vi "Convert Message Definition to Message Configuration.vi"(11 "message definition":T2={"name"="", "message type"="BC to RT", "endpoint Tx"={"terminal address"=0, "subaddress"=0}, "endpoint Rx"={"terminal address"=0, "subaddress"=0}, "create timestamp channel"=FALSE, "mode code"=0, "number of words"=0, "parameters"=[]}) -> (3 "message configuration":T1)   [LabVIEW 2020, in "AIM MIL-STD-1553 Engine.lvlib" / "Implementation.lvlib" / "Shared Resources Factory.lvclass"]
uses:
  Shared Resources Factory.lvclass
  Shared/Message Definition.ctl
  Shared/Message Type.ctl
  Shared/Terminal Endpoint.ctl
  Shared/Address.ctl
  Shared/Parameter Definition.ctl
  Custom Device/Message Configuration.ctl
  Custom Device/Custom Device.lvlib
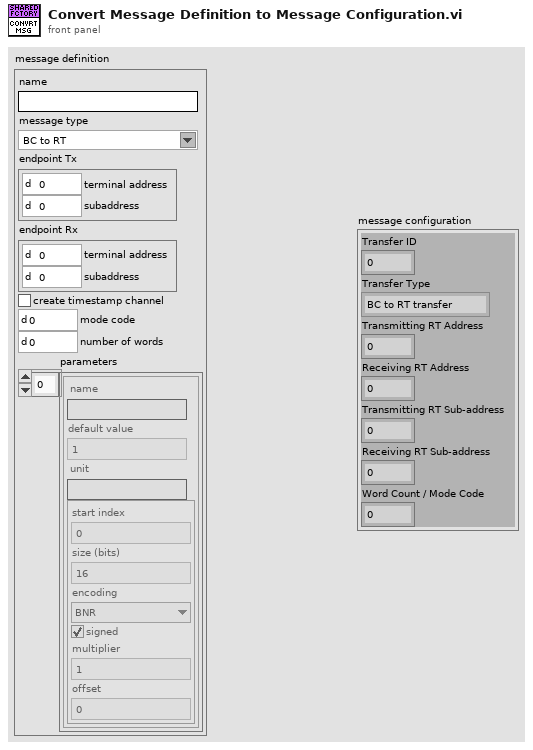
[diagram p1: front panel]
types:
  T1 = typedef "AIM MIL-STD-1553 Engine.lvlib/Custom Device.lvlib/Message Configuration.ctl" = cluster{"Transfer ID":u16, "Transfer Type":enum16{"BC to RT transfer", "RT to BC transfer", "RT to RT transfer"}, "Transmitting RT Address":u8, "Receiving RT Address":u8, "Transmitting RT Sub-address":u8, "Receiving RT Sub-address":u8, "Word Count / Mode Code":u8}
  T2 = typedef "Message Definition.ctl" = cluster{"name":string, "message type":T3, "endpoint Tx":T4, "endpoint Rx":T4, "create timestamp channel":bool, "mode code":u16, "number of words":u16, "parameters":cluster{"name":string, "default value":dbl, "unit":string, "parameter definition":T6}[]}
  T3 = typedef "Message Type.ctl" = string
  T4 = typedef "Terminal Endpoint.ctl" = cluster{"terminal address":T5, "subaddress":T5}
  T5 = typedef "Address.ctl" = u16
  T6 = typedef "Parameter Definition.ctl" = cluster{"start index":i32, "size (bits)":i32, "encoding":enum16{"BNR", "BCD", "Discrete"}, "signed":bool, "multiplier":dbl, "offset":dbl}
  T7 = enum16{"BC to RT transfer", "RT to BC transfer", "RT to RT transfer"}
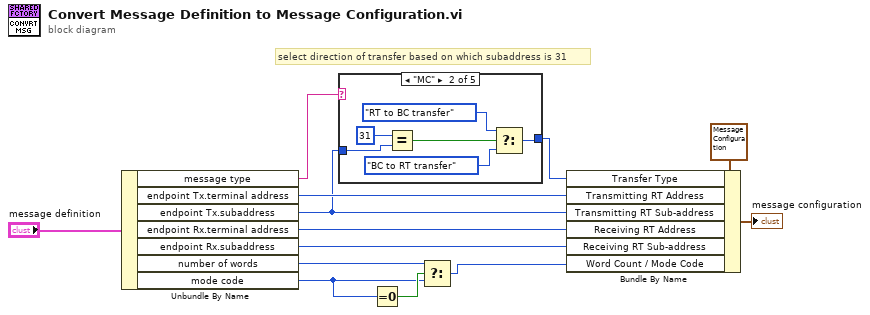
[diagram p0: block diagram]
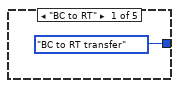
[diagram p2: hidden frame]
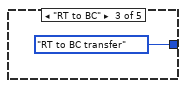
[diagram p3: hidden frame]
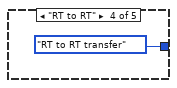
[diagram p4: hidden frame]
diagram:
  # "select direction of transfer based on which subaddress is 31"
  n1 = Unbundle By Name("message definition") -> ("message type"=w10:T3, "endpoint Tx.terminal address"=w8:T5, "endpoint Tx.subaddress"=w1:T5, "endpoint Rx.terminal address"=w7:T5, "endpoint Rx.subaddress"=w6:T5, "number of words"=w4:u16, "mode code"=w3:u16)
  n2 = case shown="\"MC\"" w10 {
    tunnel: [T7."BC to RT transfer" ("Transfer Type") w17 T7."RT to BC transfer" ("Transfer Type") T7."RT to RT transfer" ("Transfer Type") _] -> w9
    tunnel: w1 -> [_ w20 _ _ _]
    frame "BC to RT" {
    }
    frame "MC" {
      n3 = Equal?(x=T5 31, y=w20) -> (x = y?=w16:bool)
      n4 = Select(t=T7."RT to BC transfer" ("Transfer Type"), s=w16, f=T7."BC to RT transfer" ("Transfer Type")) -> (s? t:f=w17:T7)
    }
    frame "RT to BC" {
    }
    frame "RT to RT" {
    }
    frame Default {
    }
  }
  n5 = Equal To 0?(x=w3) -> (x = 0?=w5:bool)
  n6 = Select(t=w4, s=w5, f=w3) -> (s? t:f=w2:u16)
  n7 = Bundle By Name(cluster=T1 {"Transfer ID"=0, "Transfer Type"=enum."BC to RT transfer", "Transmitting RT Address"=0, "Receiving RT Address"=0, "Transmitting RT Sub-address"=0, "Receiving RT Sub-address"=0, "Word Count / Mode Code"=0} ("Message Configuration"), "Transfer Type"=w9, "Transmitting RT Address"=w8, "Transmitting RT Sub-address"=w1, "Receiving RT Address"=w7, "Receiving RT Sub-address"=w6, "Word Count / Mode Code"=w2) -> (→"message configuration":T1)
